vi "Sets and Query the Continuity Threshold.vi"(5 "Enable to Query":bool, 7 "Enable to Sets":bool, 8 "error in":errorcluster, 10 "Continuity Threshold":i16 min=0 max=1000 step=1, 11 "VISA resource name":refnum<visa-resource-name>) -> (0 "error out":errorcluster, 2 "Return the Continuity Threshold":string, 3 "VISA resource name out":refnum<visa-resource-name>)   [LabVIEW 2011, in "DMM4.lvlib"]
uses:
  <instrlib>/DMM4/DMM4.lvlib
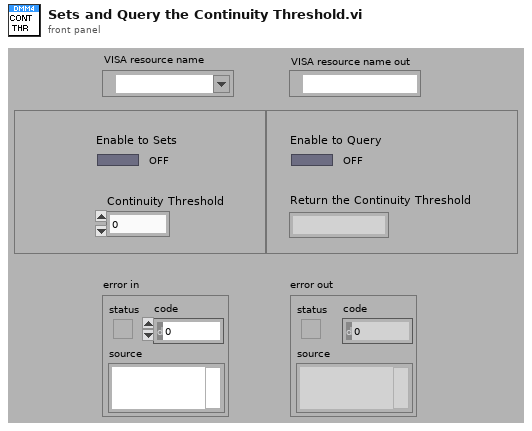
[diagram p1: front panel]
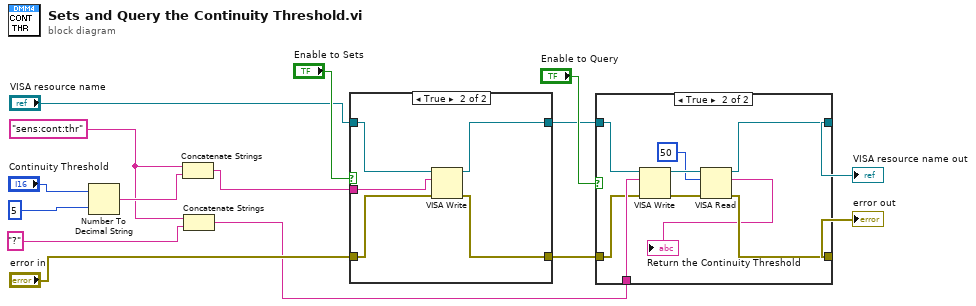
[diagram p0: block diagram]
diagram:
  w13 = "sens:cont:thr"
  n1 = Number To Decimal String(number="Continuity Threshold", width (-)=i16 5) -> (decimal integer string=w14:string)
  n2 = Concatenate Strings(w13, w14) -> (w9:string)
  n3 = Concatenate Strings(w13, "?") -> (w8:string)
  n4 = case shown="True" "Enable to Sets" {
    tunnel: "VISA resource name" -> [w17 w22]
    tunnel: "error in" -> [w16 w21]
    tunnel: [w17 w20] -> w6
    tunnel: [w16 w19] -> w5
    tunnel: w9 -> [_ w18]
    frame False {
    }
    frame True {
      n5 = VISA Write(VISA resource name=w22, write buffer=w18, error in (no error)=w21) -> (VISA resource name out=w20:refnum<visa-resource-name>, error out=w19:errorcluster)  [unwired: 1 out]
    }
  }
  n6 = case shown="True" "Enable to Query" {
    tunnel: w8 -> [_ w31]
    tunnel: w6 -> [w24 w30]
    tunnel: w5 -> [w23 w29]
    tunnel: [w24 w28] -> w4
    tunnel: [w23 w27] -> w3
    frame False {
    }
    frame True {
      n7 = VISA Write(VISA resource name=w30, write buffer=w31, error in (no error)=w29) -> (VISA resource name out=w32:refnum<visa-resource-name>, error out=w33:errorcluster)  [unwired: 1 out]
      n8 = VISA Read(VISA resource name=w32, byte count=u32 50, error in (no error)=w33) -> (VISA resource name out=w28:refnum<visa-resource-name>, read buffer=→"Return the Continuity Threshold":string, error out=w27:errorcluster)  [unwired: 1 out]
    }
  }
  "VISA resource name out" <- w4
  "error out" <- w3
